vi "ep_Windows for Speed Estimation.vi"(0 "all spectra points":cluster{"frequency":dbl[], "magnitude":dbl[]}, 1 "df":dbl format="%#_13g", 5 "fundamental frequency [Hz]":dbl format="%#_13g", 7 "nominal frequency":enum16{"50 Hz", "60 Hz"}(ring), 9 "nameplate speed":T3, 11 "error in (no error)":errorcluster) -> (4 "points in window":T1(array[cluster]), 8 "pole pairs":i32, 10 "range of speed":T2, 15 "error out":errorcluster)   [LabVIEW 2014, in "NI_EP_Motor Monitoring.lvlib"]
uses:
  <vilib>/addons/Electrical Power/Motor Monitoring/NI_EP_Motor Monitoring.lvlib
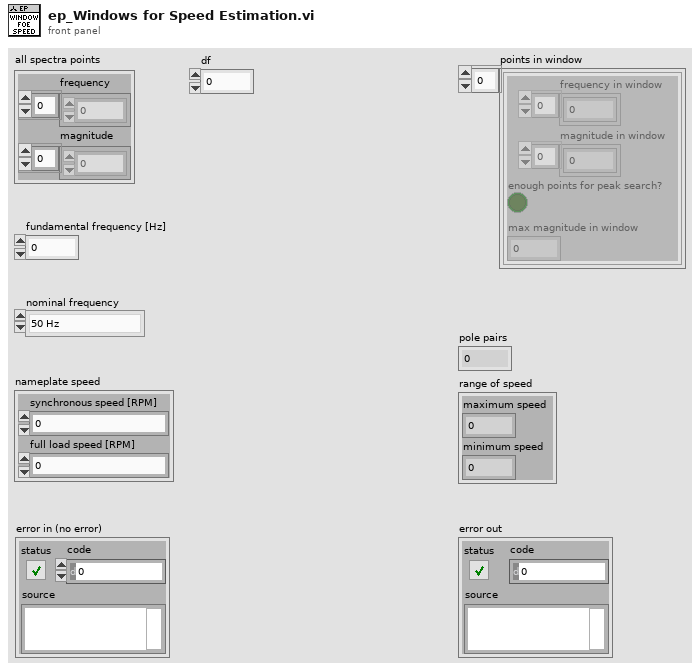
[diagram p1: front panel]
types:
  T1 = cluster{"frequency in window":dbl[], "magnitude in window":dbl[], "enough points for peak search?":bool, "max magnitude in window":dbl}[]
  T2 = cluster{"maximum speed":dbl, "minimum speed":dbl}
  T3 = cluster{"synchronous speed [RPM]":dbl, "full load speed [RPM]":dbl}
  T4 = cluster{"maximum frequency [Hz]":dbl, "slip error allowance":dbl, "minimum points for peak search":dbl, "accuracy of fs":dbl, "difference?":bool, " fs harmonics order":i32, "fs forbidden range":dbl, "p3:p1 valid significance ratio":dbl, "ratio for significance weighting":dbl, "significance weighting":dbl}
  T5 = cluster{"window2_lower":dbl, "window2_upper":dbl}
  T6 = cluster{"window1_lower":dbl, "window1_upper":dbl}
  T7 = cluster{"window3_lower":dbl, "window3_upper":dbl}
  T8 = cluster{"window4_lower":dbl, "window4_upper":dbl}
  T9 = cluster{"window4_lower":dbl, "window4_upper":dbl}[]
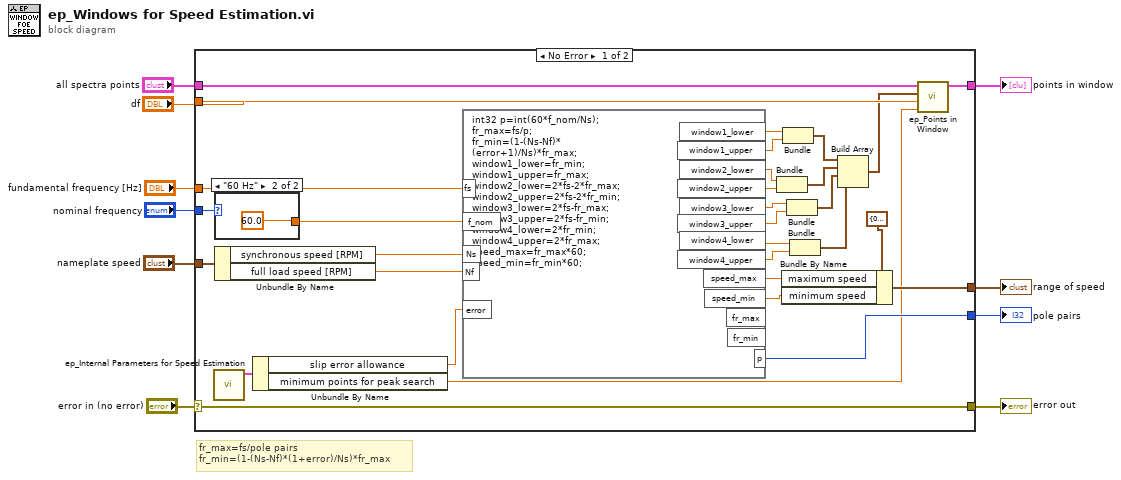
[diagram p0: block diagram]
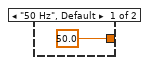
[diagram p2: hidden frame]
diagram:
  # "fr_max=fs/pole pairs\nfr_min=(1-(Ns-Nf)*(1+error)/Ns)*fr_max"
  n1 = case shown="No Error" "error in (no error)" {
    selector: "error in (no error)" -> [w11 w44]
    tunnel: "nameplate speed" -> [w41 _]
    tunnel: [w35 _] -> w10
    tunnel: "fundamental frequency [Hz]" -> [w40 _]
    tunnel: [w11 w44] -> w7
    tunnel: "nominal frequency" -> [w39 _]
    tunnel: [w31 _] -> w4
    tunnel: "all spectra points" -> [w24 _]
    tunnel: [w23 _] -> w1
    tunnel: "df" -> [w22 _]
    frame No Error {
      n2 = call <vilib>:"ep_Internal Parameters for Speed Estimation.vi"() -> ("internal parameters for speed estimation"=w21:T4)  [unwired: 11 in]
      n3 = case shown="\"60 Hz\"" w39 {
        tunnel: [50.0 60.0] -> w38
        frame "50 Hz", Default {
        }
        frame "60 Hz" {
        }
      }
      n4 = Unbundle By Name(w41) -> ("synchronous speed [RPM]"=w37:dbl, "full load speed [RPM]"=w36:dbl)
      n5 = Unbundle By Name(w21) -> ("slip error allowance"=w20:dbl, "minimum points for peak search"=w19:dbl)
      n6 = formula code="int32 p=int(60*f_nom/Ns);\nfr_max=fs/p;\nfr_min=(1-(Ns-Nf)*\n(error+1)/Ns)*fr_max;\nwindow1_lower=fr_min;\nwindow1_upper=fr_max;\nwindow2_lower=2*fs-2*fr_max;\nwindow2_upper=2*fs-2*fr_min;\nwindow3_lower=2*fs-fr_max;\nwindow3_upper=2*fs-fr_min;\nwindow4_lower=2*fr_min;\nwindow4_upper=2*fr_max;\nspeed_max=fr_max*60;\nspeed_min=fr_min*60;"("fs"=w40, "Ns"=w37, "Nf"=w36, "f_nom"=w38, "error"=w20) -> ("window1_upper"=w29:dbl, "window1_lower"=w30:dbl, "window2_upper"=w27:dbl, "window2_lower"=w28:dbl, "p"=w35:i32, "speed_max"=w33:dbl, "speed_min"=w34:dbl, "window3_lower"=w17:dbl, "window3_upper"=w15:dbl, "window4_lower"=w13:dbl, "window4_upper"=w14:dbl)  [unwired: 2 out]
      n7 = Bundle("window2_lower"=w28, "window2_upper"=w27) -> (w25:T5)  [unwired: 1 in]
      n8 = Bundle By Name(cluster=T2 {"maximum speed"=0.0, "minimum speed"=0.0}, "maximum speed"=w33, "minimum speed"=w34) -> (w31:T2)
      n9 = Bundle("window1_lower"=w30, "window1_upper"=w29) -> (w26:T6)  [unwired: 1 in]
      n10 = Bundle("window3_lower"=w17, "window3_upper"=w15) -> (w16:T7)  [unwired: 1 in]
      n11 = Bundle("window4_lower"=w13, "window4_upper"=w14) -> (w12:T8)  [unwired: 1 in]
      n12 = Build Array(w26, w25, w16, w12) -> (w18:T9)
      n13 = call <vilib>:"ep_Points in Window.vi"("minimum points for peak search"=w19, "df"=w22, "window configuration"=w18, "all spectra points"=w24) -> ("points in window"=w23:T1)  [unwired: 7 in]
    }
    frame Error {
    }
  }
  "error out" <- w7
  "pole pairs" <- w10
  "range of speed" <- w4
  "points in window" <- w1
